vi "setPhase.vi"(7 "Channel":string="0", 8 "error in (no error)":errorcluster, 10 "Phase [°]":dbl, 11 "FgenKeysight in":refnum<class "ArbKeysight.lvclass">) -> (0 "error out":errorcluster, 3 "FgenKeysight out":refnum<class "ArbKeysight.lvclass">)   [LabVIEW 2023, in "ArbKeysight.lvclass"]
doc: "<b>Author:</b> Wolfgang\n<b>Description:</b> Set Output Phase in degree"
uses:
  ArbKeysight.lvclass
  ArbKeysight.lvclass/ArbKeysight.ctl
  Arb.lvclass
  Driver/Keysight-33500B.lvlib
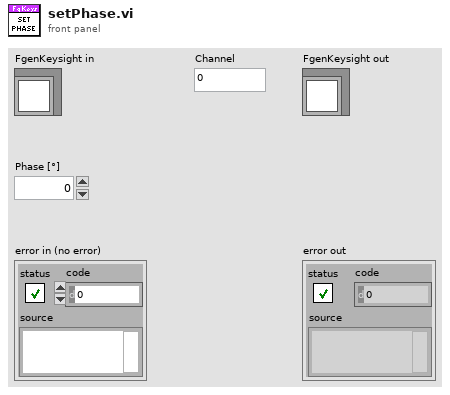
[diagram p1: front panel]
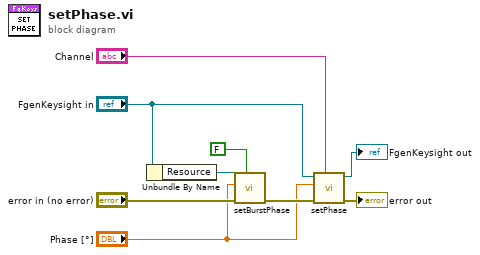
[diagram p0: block diagram]
diagram:
  n1 = Unbundle By Name("FgenKeysight in") -> ("Resource"=w3:refnum<visa-resource-name>)
  n2 = call "setBurstPhase.vi"("Burst"=FALSE, "error in (no error)"="error in (no error)", "Phase"="Phase [°]", "VISA resource name"=w3) -> ("error out"=w5:errorcluster)  [unwired: 6 in, 1 out]
  n3 = call-parent "setPhase.vi"("Channel"="Channel", "error in (no error)"=w5, "Phase [°]"="Phase [°]", "Fgen in"="FgenKeysight in") -> ("error out"=→"error out":errorcluster, "Fgen out"=→"FgenKeysight out":refnum<class "ArbKeysight.lvclass">)  [unwired: 6 in]
